vi "test direct summing.vi"() -> ()   [LabVIEW 2015]
panel:
  in  "Two Cameras?":bool
  out "XY Graph":cluster{dbl[], dbl[]}[](graph)
  in  "Na / Rb":u16(ring) items=["Na", "Rb"]
  in  "Fitting Results Save Path":string
  in  "Best Fit Parameters":dbl[](array[numeric])
  in  "Image Data":dbl[][](array[numeric])
  in  "Fitting Type":u16(ring) items=["2D Gaussian", "2D Quadraple", "Double Gaussian", "Double Quadraple", "Triple Gaussian"]
  in  "File Num":u16
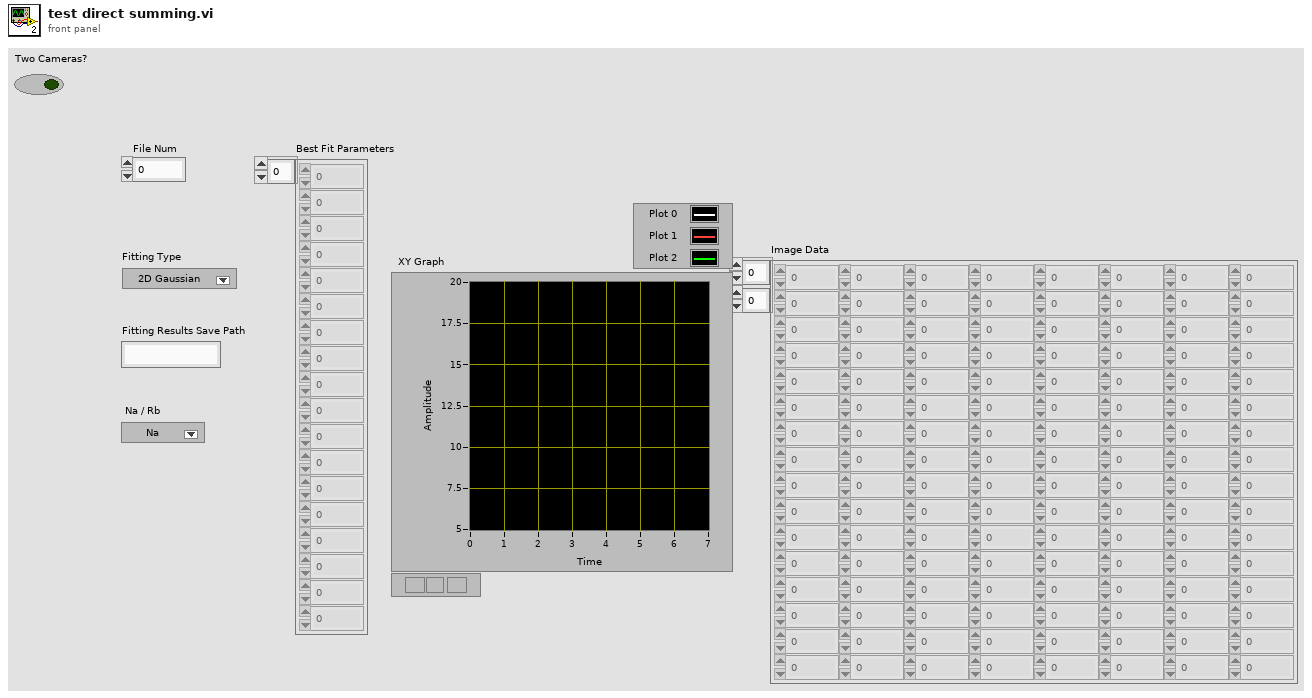
[diagram p1: front panel]
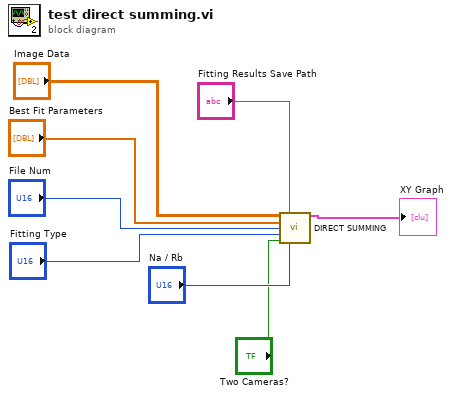
[diagram p0: block diagram]
diagram:
  n1 = call "DIRECT SUMMING.vi"("Image Data"="Image Data", "Fitting Results Save Path"="Fitting Results Save Path", "Best Fit Parameters"="Best Fit Parameters", "File Num"="File Num", "Fitting Type"="Fitting Type", "Two Cameras?"="Two Cameras?", "Na / Rb"="Na / Rb") -> ("XY Graph"=→"XY Graph":cluster{dbl[], dbl[]}[])  [unwired: 8 in]
